vi "CreateBrowerComponent.vi"(8 "error in (no error)":errorcluster, 10 "SymbolIndex":i32, 11 "BrowerBrowerFactory in":refnum<class "BrowerFactory.lvclass">) -> (0 "error out":errorcluster, 2 "BrowerComponent":refnum<class "BrowerComponent.lvclass">, 3 "BrowerBrowerFactory out":refnum<class "BrowerFactory.lvclass">)   [LabVIEW 2015, in "BrowerFactory.lvclass"]
uses:
  BrowerFactory.lvclass
  BrowerComponent/BrowerComponent/BrowerComponent.lvclass
  BrowerComponent/BrowerComposite/BrowerComposite.lvclass
  BrowerComponent/BrowerLeaf/BrowerLeaf.lvclass
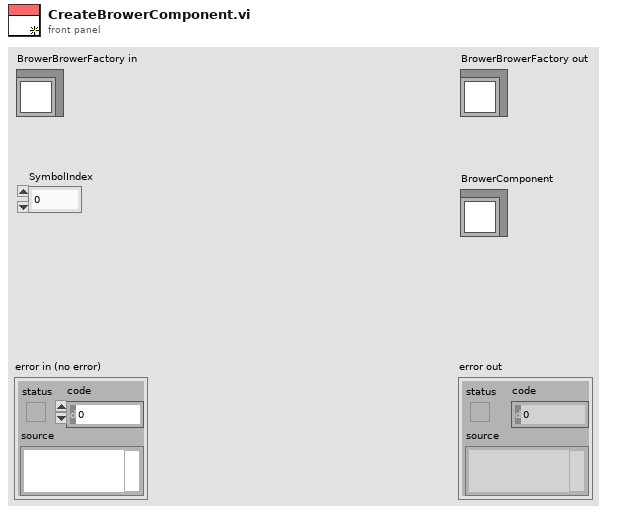
[diagram p1: front panel]
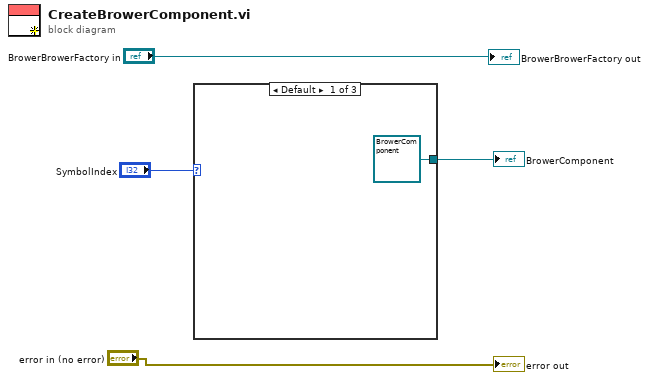
[diagram p0: block diagram]
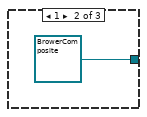
[diagram p2: hidden frame]
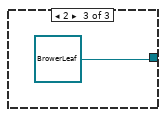
[diagram p3: hidden frame]
diagram:
  n1 = case shown="Default" "SymbolIndex" {
    tunnel: [refnum<class "BrowerComponent.lvclass"> refnum ("BrowerLeaf") refnum<class "BrowerComposite.lvclass"> refnum ("BrowerComposite") refnum<class "BrowerLeaf.lvclass"> refnum ("BrowerLeaf")] -> w1
    frame Default {
    }
    frame 1 {
    }
    frame 2 {
    }
  }
  "BrowerComponent" <- w1
  "error out" <- "error in (no error)"
  "BrowerBrowerFactory out" <- "BrowerBrowerFactory in"
